vi "Disconnect.vi"(8 "error in":errorcluster, 11 "4322 in":refnum<class "4322.lvclass">) -> (0 "error out":errorcluster, 3 "4322 out":refnum<class "4322.lvclass">)   [LabVIEW 2019, in "4322.lvlib" / "4322.lvclass"]
uses:
  Library/4322.lvclass
  Library/4322.lvclass/4322.ctl
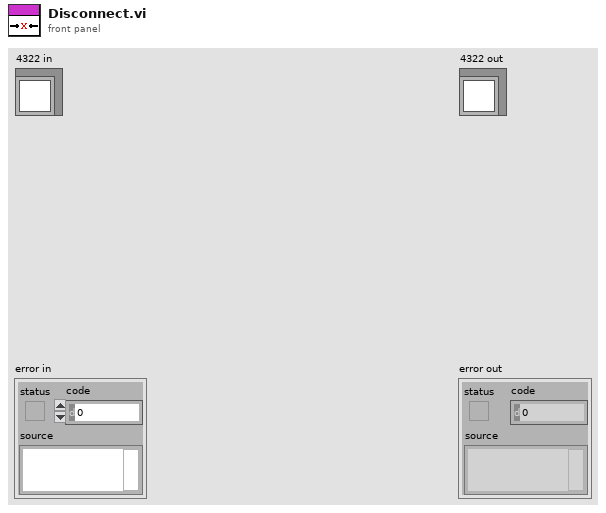
[diagram p1: front panel]
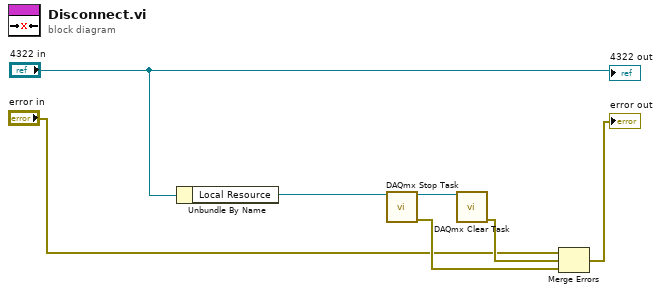
[diagram p0: block diagram]
diagram:
  n1 = Unbundle By Name("4322 in") -> ("Local Resource"=w7:refnum<k21>)
  n2 = call <vilib>:"DAQmx Stop Task.vi"("task/channels in"=w7) -> ("task out"=w6:refnum<k21>, "error out"=w5:errorcluster)  [unwired: 13 in]
  n3 = call <vilib>:"DAQmx Clear Task.vi"("task in"=w6) -> ("error out"=w4:errorcluster)  [unwired: 14 in]
  n4 = Merge Errors("error in", w4, w5) -> (→"error out":errorcluster)
  "4322 out" <- "4322 in"
